vi "Extract time from string.vi"(0 "ics time string":string, 11 "Error In":errorcluster) -> (4 "Time and Date":timestamp, 15 "Error Out":errorcluster)   [LabVIEW 2020]
doc: "Extract time from string VI extracts time from ics format string."
uses:
  <vilib>/Utility/miscctls.llb/LVDateTimeRec.ctl
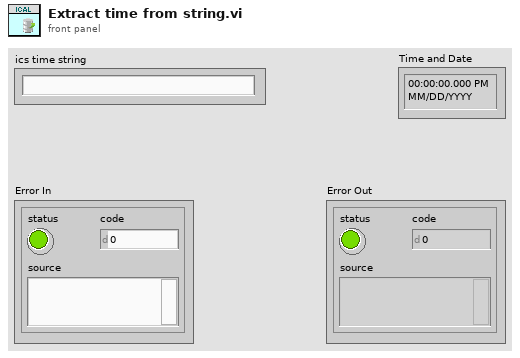
[diagram p1: front panel]
types:
  T1 = typedef "LVDateTimeRec.ctl" = cluster{"fractional second":dbl, "second":i32, "minute":i32, "hour":i32, "day of month":i32, "month":i32, "year":i32, "day of week":i32, "day of year":i32, "DST":i32}
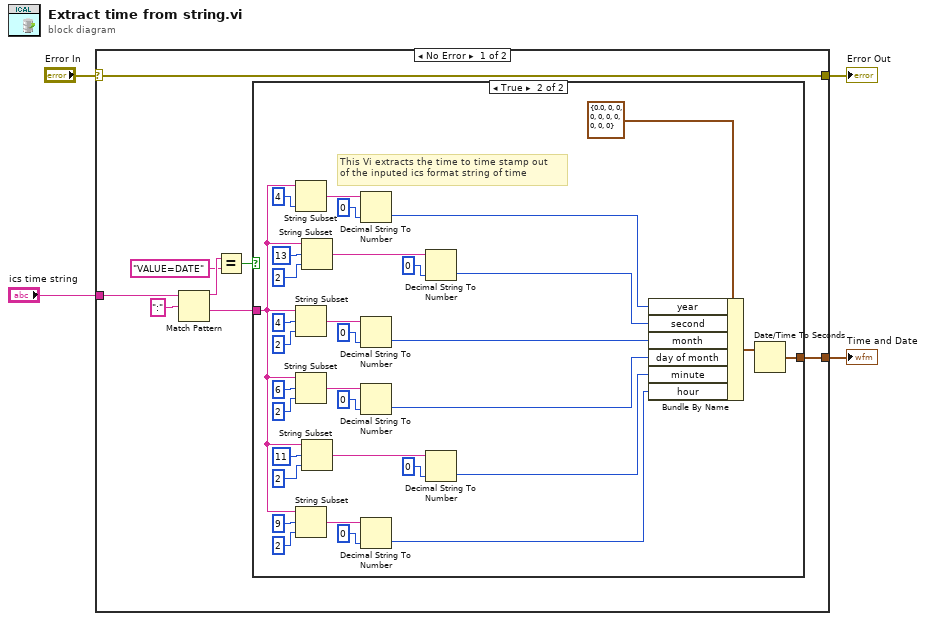
[diagram p0: block diagram]
diagram:
  n1 = case shown="No Error" "Error In" {
    selector: "Error In" -> [w12 w46]
    tunnel: [w12 w46] -> w3
    tunnel: "ics time string" -> [w9 _]
    tunnel: [w7 _] -> w1
    frame No Error {
      n2 = Match Pattern(string=w9, regular expression=":") -> (before substring=w11:string, after substring=w5:string)  [unwired: 1 in, 2 out]
      n3 = Equal?(x=w11, y="VALUE=DATE") -> (x = y?=w6:bool)
      n4 = case shown="True" w6 {
        tunnel: w5 -> [_ w14]
        tunnel: [_ w13] -> w7
        frame False {
        }
        frame True {
          # "This Vi extracts the time to time stamp out \nof the inputed ics format string of time"
          n5 = String Subset(string=w14, length (rest)=4 ("length (rest)")) -> (substring=w20:string)  [unwired: 1 in]
          n6 = String Subset(string=w14, offset (0)=4, length (rest)=2 ("length (rest)")) -> (substring=w19:string)
          n7 = String Subset(string=w14, offset (0)=6, length (rest)=2 ("length (rest)")) -> (substring=w18:string)
          n8 = String Subset(string=w14, offset (0)=9, length (rest)=2 ("length (rest)")) -> (substring=w21:string)
          n9 = String Subset(string=w14, offset (0)=13, length (rest)=2 ("length (rest)")) -> (substring=w40:string)
          n10 = String Subset(string=w14, offset (0)=11, length (rest)=2 ("length (rest)")) -> (substring=w23:string)
          n11 = Decimal String To Number(string=w20, default (0L)=0 ("Hours")) -> (number=w44:i32)  [unwired: 1 in, 1 out]
          n12 = Decimal String To Number(string=w19, default (0L)=0 ("Hours")) -> (number=w41:i32)  [unwired: 1 in, 1 out]
          n13 = Decimal String To Number(string=w18, default (0L)=0 ("Hours")) -> (number=w42:i32)  [unwired: 1 in, 1 out]
          n14 = Decimal String To Number(string=w21, default (0L)=0 ("Hours")) -> (number=w15:i32)  [unwired: 1 in, 1 out]
          n15 = Decimal String To Number(string=w40, default (0L)=0 ("Hours")) -> (number=w17:i32)  [unwired: 1 in, 1 out]
          n16 = Decimal String To Number(string=w23, default (0L)=0 ("Hours")) -> (number=w16:i32)  [unwired: 1 in, 1 out]
          n17 = Bundle By Name(cluster=T1 {"fractional second"=0.0, "second"=0, "minute"=0, "hour"=0, "day of month"=0, "month"=0, "year"=0, "day of week"=0, "day of year"=0, "DST"=0} ("date time rec"), "year"=w44, "second"=w17, "month"=w41, "day of month"=w42, "minute"=w16, "hour"=w15) -> (w45:T1)
          n18 = Date/Time To Seconds(2:w45) -> (0:w13:timestamp)  [unwired: 1 in]
        }
      }
    }
    frame Error {
    }
  }
  "Error Out" <- w3
  "Time and Date" <- w1
